vi "DCS_Noise_Check.vi"(11 "8 DCS Waveforms":dbl[][](array[numeric])) -> (3 "Boolean":bool)   [LabVIEW 2015]
doc: "Takes each channel and determines if the max value sufficiently exceeds the noise. \"Noise Factor\" is hard coded based on obseved DCS behavior. This returns a boolean in order to determine if there is in fact a signal."
uses:
  <vilib>/Analysis/NI_AALBase.lvlib
panel:
  in  "Noise Factor":dbl=6.0
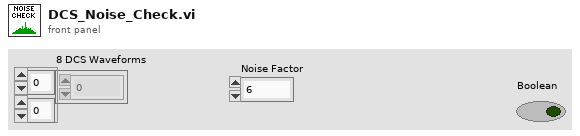
[diagram p1: front panel]
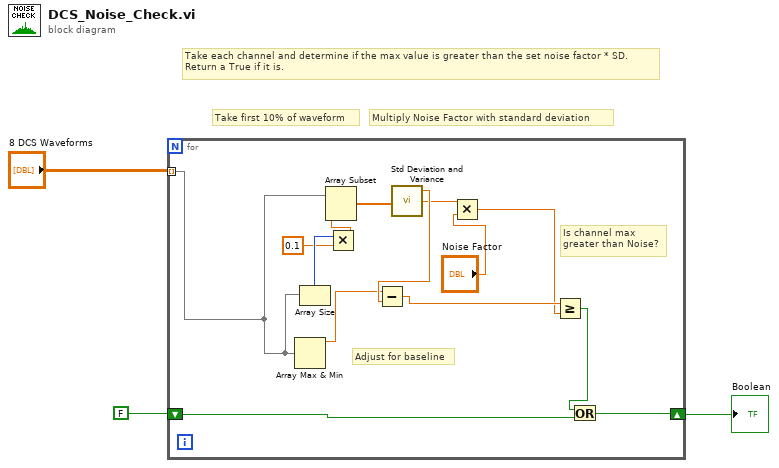
[diagram p0: block diagram]
diagram:
  # "Multiply Noise Factor with standard deviation"
  # "Take first 10% of waveform"
  # "Take each channel and determine if the max value is greater than the set noise factor * SD.\nReturn a True if it is."
  n1 = for {
    tunnel: "8 DCS Waveforms" -> [w12] mode=indexing
    shift-right: [w17] -> w1
    shift-left: FALSE ("Boolean 2") -> [w16]
    # "Is channel max\ngreater than Noise?"
    # "Adjust for baseline"
    n2 = Array Max & Min(array=w12) -> (max value=w9:dbl)  [unwired: 3 out]
    n3 = Array Size(array=w12) -> (size(s)=w15:i32)
    n4 = Multiply(x=w15, y=0.1) -> (x*y=w13:dbl)
    n5 = Array Subset(array=w12, length=w13) -> (w11:dbl[])  [unwired: 1 in]
    n6 = call <vilib>:"Std Deviation and Variance.vi"("X"=w11) -> ("mean"=w10:dbl, "standard deviation"=w7:dbl)  [unwired: 1 in, 1 out]
    n7 = Subtract(x=w9, y=w10) -> (x-y=w8:dbl)
    n8 = Multiply(x=w7, y="Noise Factor") -> (x*y=w5:dbl)
    n9 = Greater Or Equal?(x=w8, y=w5) -> (x >= y?=w4:bool)
    n10 = Or(x=w4, y=w16) -> (x .or. y?=w17:bool)
  }
  "Boolean" <- w1
